vi "Dut Close.vi"(0 "MTK7615 in":refnum<class "MTK7615.lvclass">, 11 "error in (no error)":errorcluster) -> (4 "MTK7615 out":refnum<class "MTK7615.lvclass">, 15 "error out":errorcluster)   [LabVIEW 2015, in "MTK7615.lvlib" / "MTK7615.lvclass"]
uses:
  MTK7615.lvclass
  MTK7615.lvclass/MTK7615.ctl
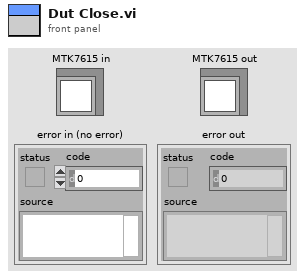
[diagram p1: front panel]
types:
  T1 = typedef "niDCT_TELNET_PrivRef.ctl" = refnum<data-value>
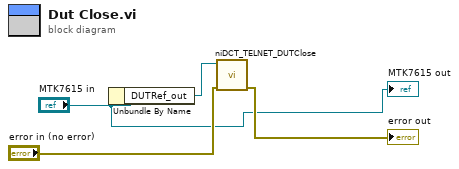
[diagram p0: block diagram]
diagram:
  n1 = Unbundle By Name("MTK7615 in") -> ("DUTRef_out"=w4:T1)
  n2 = call "niDCT_TELNET_DUTClose.vi"("error in (no error)"="error in (no error)", "DUTRef"=w4) -> ("error out"=→"error out":errorcluster)  [unwired: 9 in]
  "MTK7615 out" <- "MTK7615 in"
